vi "save stim message.vi"   [LabVIEW 2012]
panel:
  # "Stim Protocol saved"
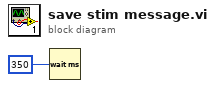
[diagram p0: block diagram]
diagram:
  n1 = Wait (ms)(milliseconds to wait=u32 350) -> ()  [unwired: 1 out]
